vi "estesiquesi.vi"() -> ()   [LabVIEW 2017]
doc: "The myRIO Project template acquires acceleration data from the onboard accelerometer and displays the changes of acceleration values in a waveform chart."
panel:
  in  "Calibrar":bool
  in  "Home":bool
  in  "Ir_posicion":bool
  in  "Fijar Posición":dbl
  out "Posición en X":dbl
  in  "Abajo_X":bool
  in  "Arriba_X":bool
  in  "Avance":dbl
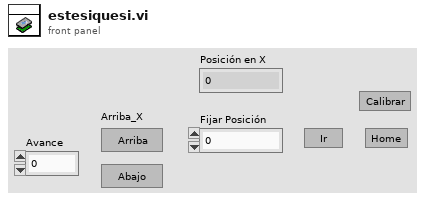
[diagram p1: front panel]
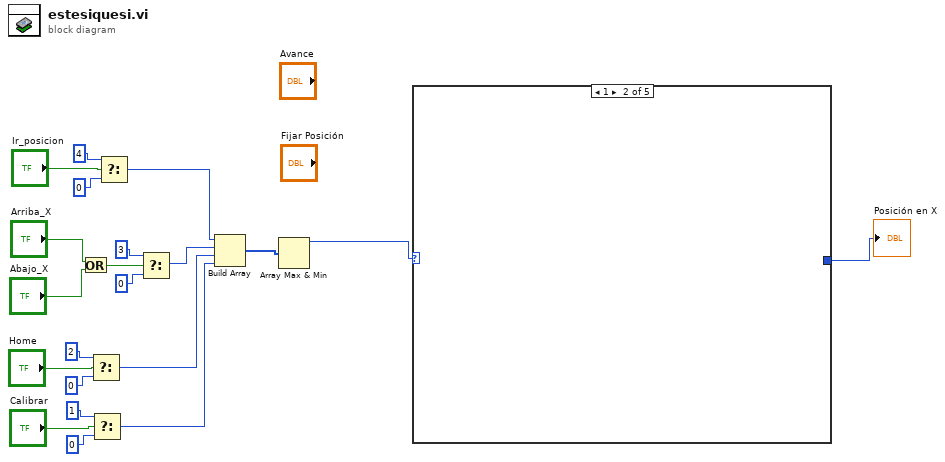
[diagram p0: block diagram]
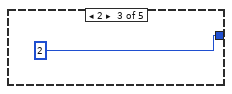
[diagram p3: hidden frame]
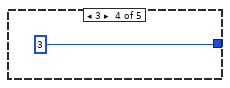
[diagram p4: hidden frame]
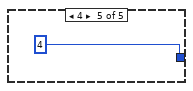
[diagram p5: hidden frame]
diagram:
  n1 = Or(x="Arriba_X", y="Abajo_X") -> (x .or. y?=w9:bool)
  n2 = Select(t=2, s="Home", f=0) -> (s? t:f=w5:i32)
  n3 = Select(t=1, s="Calibrar", f=0) -> (s? t:f=w4:i32)
  n4 = Select(t=4, s="Ir_posicion", f=0) -> (s? t:f=w7:i32)
  n5 = Select(t=3, s=w9, f=0) -> (s? t:f=w6:i32)
  n6 = Build Array(w7, w6, w5, w4) -> (w3:i32[])
  n7 = Array Max & Min(array=w3) -> (max value=w2:i32)  [unwired: 3 out]
  n8 = case shown="1" w2 {
    tunnel: [_ _ 2 3 4] -> w1
    frame 0, Default {
    }
    frame 1 {
    }
    frame 2 {
    }
    frame 3 {
    }
    frame 4 {
    }
  }
  "Posición en X" <- w1
